vi "tm_errorreport.vi"(1 "Source":path, 2 "Error":u32) -> (0 "error out":errorcluster {"code" format="%.0x"})   [LabVIEW 2023]
uses:
  tmcamcon.dll
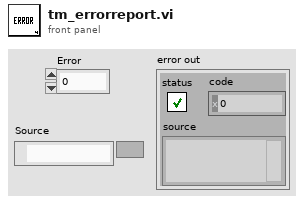
[diagram p1: front panel]
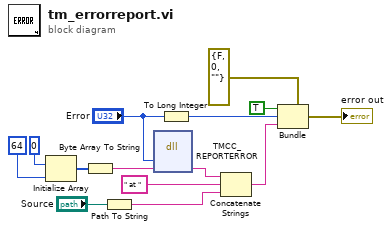
[diagram p0: block diagram]
diagram:
  n1 = Initialize Array(u8 0, 64) -> (w4:u8[])
  n2 = Byte Array To String(unsigned byte array=w4) -> (string=w1:string)
  n3 = Path To String(path="Source") -> (string=w10:string)
  n4 = dll-call lib="tmcamcon.dll" fn="TMCC_REPORTERROR"("error"="Error", "message"=w1) -> ("message"=w7:string)  [unwired: 5 in, 2 out]
  n5 = To Long Integer(number="Error") -> (32bit integer=w5:i32)
  n6 = Concatenate Strings(w7, " at ", w10) -> (w9:string)
  n7 = Bundle(cluster=cluster{"status":bool, "Erval":i32, string} {"status"=FALSE, "Erval"=0, ""}, "status"=TRUE, "Erval"=w5, w9) -> (→"error out":cluster{"status":bool, "Erval":i32, string})
